vi "Send Message.vi"(7 "Response Type (None)":refnum<class "Response.lvclass">, 8 "error in (no error)":errorcluster, 9 "timeout in ms (1000)":i32=1000, 10 "Client Message":refnum<class "Client Message.lvclass">, 11 "OBS in":refnum<class "OBS.lvclass">) -> (0 "error out":errorcluster, 1 "Has Response?":bool, 2 "Response":refnum<class "Response.lvclass">, 3 "OBS out":refnum<class "OBS.lvclass">)   [LabVIEW 2020, in "obs-websocket.lvlib" / "OBS.lvclass"]
uses:
  OBS.lvclass
  OBS.lvclass/OBS.ctl
  Client Message/Client Message.lvclass
  Client Message.ctl
  lv-promises/Promises/Promise/Promise.lvclass
  Response/Response.lvclass
  C:/dev/lv20CE/relink/lv-obs-websocket/obs-websocket/Server Message/Server Message.lvclass
  C:/dev/lv20CE/relink/lv-obs-websocket/obs-websocket/Message/Message.lvclass
  C:/dev/lv20CE/relink/lv-obs-websocket/obs-websocket/Response/Response.lvclass
  C:/dev/lv20CE/relink/lv-promises/Promises/Value/Value.lvclass
  lv-promises/Promises/Future/Future.lvclass
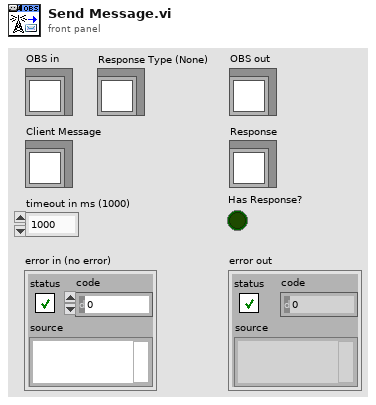
[diagram p1: front panel]
types:
  T1 = typedef "obs-websocket.lvlib/OBS.lvclass/Client Message.ctl" = cluster{"Message":refnum<class "Client Message.lvclass">, "Promise":refnum<class "Promise.lvclass">}
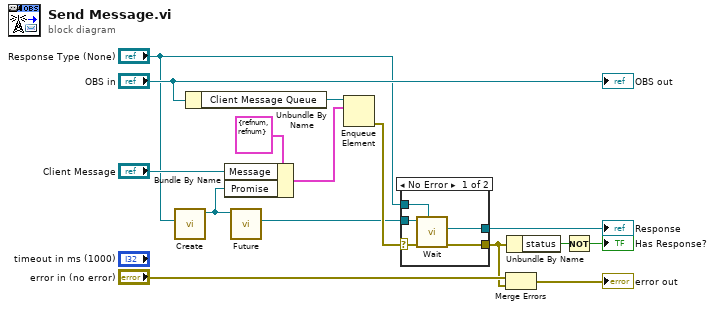
[diagram p0: block diagram]
diagram:
  n1 = call "Create.vi"("Result Type"="Response Type (None)") -> ("Promise"=w6:refnum<class "Promise.lvclass">)  [unwired: 9 in, 1 out]
  n2 = Unbundle By Name("OBS in") -> ("Client Message Queue"=w8:refnum<queue>)
  n3 = Bundle By Name(cluster=T1 {"Message"=refnum, "Promise"=refnum} ("Client Message"), "Message"="Client Message", "Promise"=w6) -> (w7:T1)
  n4 = call "Future.vi"("Promise in"=w6) -> ("Future"=w5:refnum<class "Future.lvclass">)  [unwired: 9 in, 1 out]
  n5 = Enqueue Element(queue=w8, element=w7) -> (error out=w15:errorcluster)  [unwired: 2 in, 2 out]
  n6 = case shown="No Error" w15 {
    selector: w15 -> [w20 w21]
    tunnel: w5 -> [w19 _]
    tunnel: "Response Type (None)" -> [w18 w22]
    tunnel: [w17 w22] -> w3
    tunnel: [w16 w21] -> w1
    frame No Error {
      n7 = call "Wait.vi"("Result Type"=w18, "error in (no error)"=w20, "Future in"=w19) -> ("error out"=w16:errorcluster, "Result"=w17:refnum<class "Response.lvclass">)  [unwired: 7 in]
    }
    frame Error {
    }
  }
  "Response" <- w3
  n8 = Merge Errors("error in (no error)", w1) -> (→"error out":errorcluster)
  n9 = Unbundle By Name(w1) -> ("status"=w2:bool)
  n10 = Not(x=w2) -> (.not. x?=→"Has Response?":bool)
  "OBS out" <- "OBS in"
